vi "Global_simulator.vi"() -> ()   [LabVIEW 2017]
panel:
  out "2":bool
  out "1":bool
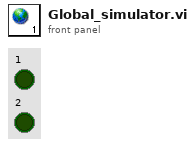
[diagram p1: front panel]
diagram:
